vi "testingstuff.vi"() -> ()   [LabVIEW 2009]
panel:
  in  "Array 2":bool[](array[boolean])
  out "Array":bool[](array[boolean])
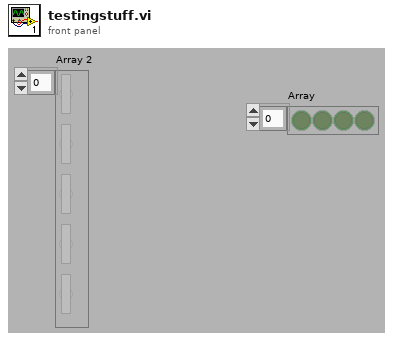
[diagram p1: front panel]
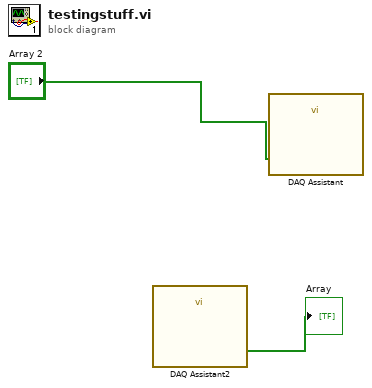
[diagram p0: block diagram]
diagram:
  n1 = call "DAQ Assistant2"() -> ("data"=→"Array":bool[])  [unwired: 17 in, 2 out]
  n2 = call "DAQ Assistant"("data"="Array 2") -> ()  [unwired: 17 in, 2 out]
